vi "visualize alignment on RGB image.vi"(8 "error in (no error)":errorcluster, 11 "Cascade in":refnum<class "Cascade.lvclass">) -> (0 "error out":errorcluster, 3 "Cascade out":refnum<class "Cascade.lvclass">)   [LabVIEW 2012, in "Cascade.lvclass"]
uses:
  Cascade.lvclass
  Cascade.lvclass/Cascade.ctl
  <vilib>/vision/NI_Vision_Development_Module.lvlib
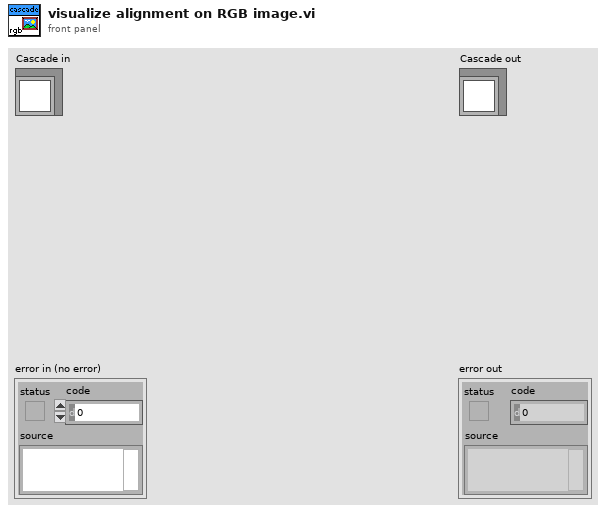
[diagram p1: front panel]
types:
  T1 = typedef "IMAQ Image.ctl" = refnum<image>
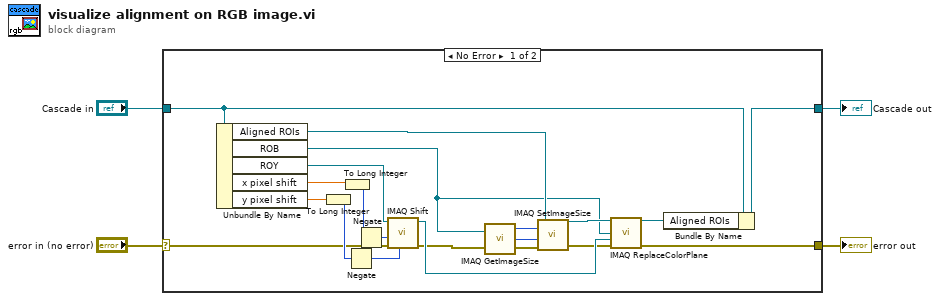
[diagram p0: block diagram]
diagram:
  n1 = case shown="No Error" "error in (no error)" {
    selector: "error in (no error)" -> [w21 w27]
    tunnel: [w20 w27] -> w3
    tunnel: [w16 w26] -> w1
    tunnel: "Cascade in" -> [w17 w26]
    frame No Error {
      n2 = Unbundle By Name(w17) -> ("Aligned ROIs"=w12:T1, "ROB"=w10:T1, "ROY"=w19:T1, "x pixel shift"=w25:dbl, "y pixel shift"=w23:dbl)
      n3 = To Long Integer(number=w23) -> (32bit integer=w22:i32)
      n4 = To Long Integer(number=w25) -> (32bit integer=w24:i32)
      n5 = Negate(x=w22) -> (-x=w13:i32)
      n6 = Negate(x=w24) -> (-x=w14:i32)
      n7 = call "IMAQ Shift"("YOffset"=w13, "error in (no error)"=w21, "XOffset"=w14, "Image Src"=w19) -> ("error out"=w6:errorcluster, "Image Dst Out"=w18:T1)  [unwired: 6 in]
      n8 = call "IMAQ GetImageSize"("Image"=w10, "error in (no error)"=w6) -> ("Y Resolution"=w8:i32, "X Resolution"=w9:i32, "error out"=w7:errorcluster)  [unwired: 2 in]
      n9 = call "IMAQ SetImageSize"("error in (no error)"=w7, "Y Resolution"=w8, "X Resolution"=w9, "Image"=w12) -> ("error out"=w5:errorcluster, "Image Out"=w11:T1)  [unwired: 1 in]
      n10 = call "IMAQ ReplaceColorPlane"("Image Src"=w11, "Red or Hue Plane"=w10, "Green or Sat Plane"=w18, "error in (no error)"=w5) -> ("Image Dst Out"=w15:T1, "error out"=w20:errorcluster)  [unwired: 10 in]
      n11 = Bundle By Name(cluster=w17, "Aligned ROIs"=w15) -> (w16:refnum<class "Cascade.lvclass">)
    }
    frame Error {
    }
  }
  "error out" <- w3
  "Cascade out" <- w1
